vi "Read from EDS file.vi"(8 "error in (no error)":errorcluster, 10 "Clust Refnum":refnum<vi>, 11 "EDS File Path":path) -> (0 "error out":errorcluster)   [LabVIEW 2013]
uses:
  <vilib>/Utility/config.llb/NI_LVConfig.lvlib
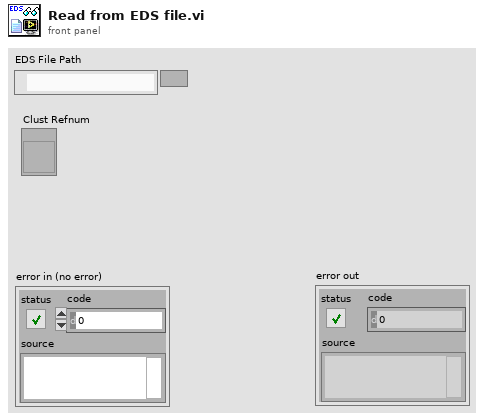
[diagram p1: front panel]
types:
  T1 = typedef "NI_LVConfig.lvlib/Config Data RefNum.ctl" = refnum<k1>
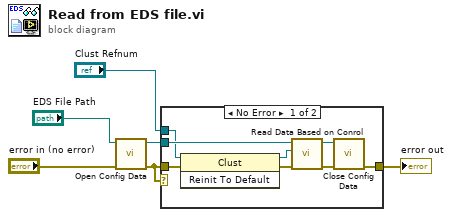
[diagram p0: block diagram]
diagram:
  n1 = call <vilib>:"Open Config Data.vi"("error in (no error)"="error in (no error)", "configuration file path"="EDS File Path") -> ("error out"=w1:errorcluster, "refnum"=w5:T1)  [unwired: 7 in, 1 out]
  n2 = case shown="No Error" w1 {
    tunnel: w5 -> [w14 _]
    tunnel: [w13 w15] -> w4
    tunnel: "Clust Refnum" -> [w10 _]
    tunnel: w1 -> [w8 w15]
    frame No Error {
      n3 = invoke on="Invoke Node" class="Clust" method="Reinit To Default"(reference=w10, error in=w8) -> (reference out=w9:refnum<vi>, error out=w7:errorcluster)  [unwired: 1 in, 1 out]
      n4 = call "Read Data Based on Conrol.vi"("error in (no error)"=w7, "Data Refnum"=w9, "File Refnum"=w14) -> ("error out"=w12:errorcluster, "dup File Refnum"=w11:T1)  [unwired: 7 in]
      n5 = call <vilib>:"Close Config Data.vi"("error in (no error)"=w12, "refnum"=w11) -> ("error out"=w13:errorcluster)  [unwired: 8 in, 1 out]
    }
    frame Error {
    }
  }
  "error out" <- w4
